vi "Handle URL.vi"(8 "error in (no error)":errorcluster, 10 "URL":string, 11 "FTP in":refnum<class "FTP.lvclass">) -> (0 "error out":errorcluster, 1 "directory":string, 2 "address":string, 3 "FTP out":refnum<class "FTP.lvclass">)   [LabVIEW 2017, in "FTP.lvlib" / "FTP.lvclass"]
uses:
  FTP.lvclass
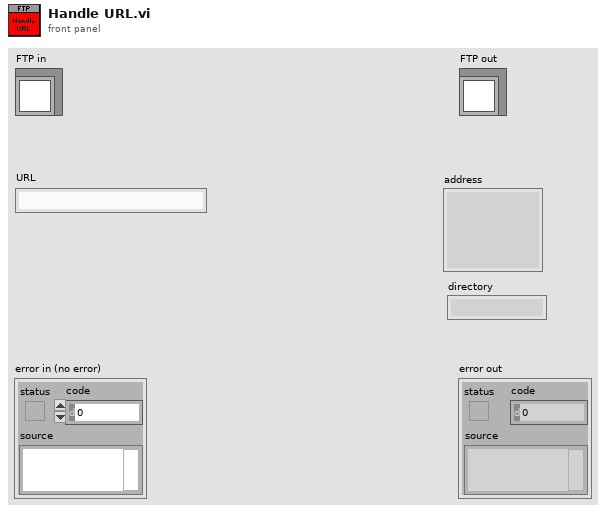
[diagram p1: front panel]
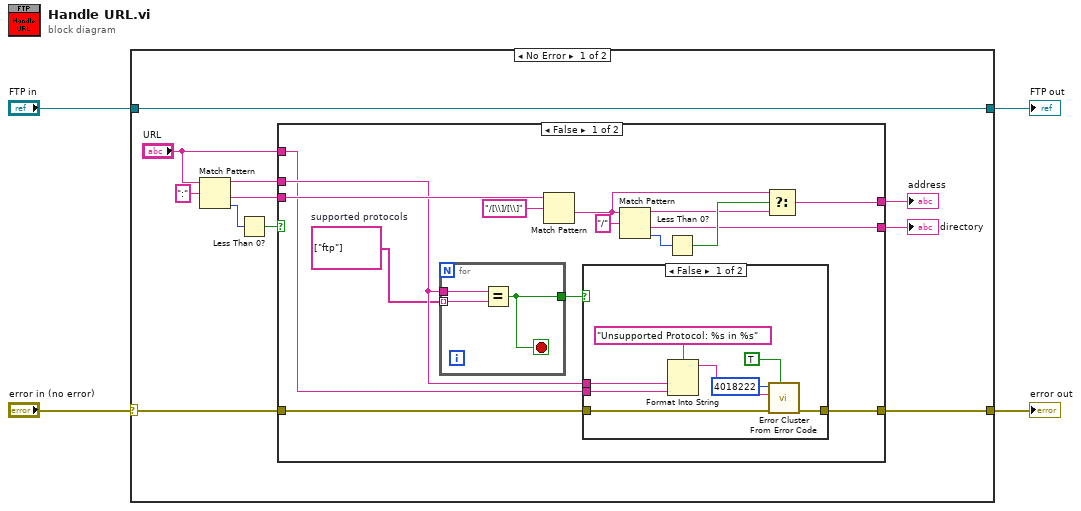
[diagram p0: block diagram]
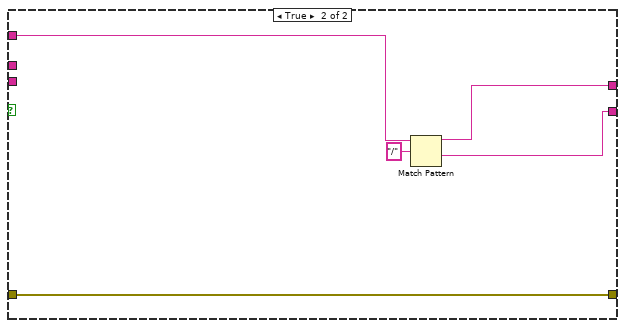
[diagram p3: hidden frame]
diagram:
  n1 = case shown="No Error" "error in (no error)" {
    selector: "error in (no error)" -> [w7 w49]
    tunnel: [w6 w49] -> w3
    tunnel: [w15 w48] -> w1
    tunnel: "FTP in" -> [w15 w48]
    frame No Error {
      n2 = Match Pattern(string="URL", regular expression=":") -> (before substring=w8:string, after substring=w12:string, offset past match=w13:i32)  [unwired: 1 in, 1 out]
      n3 = Less Than 0?(x=w13) -> (x < 0?=w10:bool)
      n4 = case shown="False" w10 {
        tunnel: w12 -> [w30 _]
        tunnel: [w18 w43] -> w11
        tunnel: "URL" -> [w25 w45]
        tunnel: w8 -> [w26 _]
        tunnel: w7 -> [w28 w47]
        tunnel: [w27 w47] -> w6
        tunnel: [w16 w44] -> w5
        frame False {
          w24 = string[] ["ftp"]  # supported protocols
          n5 = for {
            tunnel: w26 -> [w33]
            tunnel: w24 -> [w32] mode=indexing
            tunnel: [w31] -> w23
            stop <- w31 stop-if-true
            n6 = Equal?(x=w33, y=w32) -> (x = y?=w31:bool)
          }
          n7 = Match Pattern(string=w30, regular expression="/[\\]/[\\]") -> (after substring=w20:string)  [unwired: 1 in, 3 out]
          n8 = case shown="False" w23 {
            tunnel: w28 -> [w41 w42]
            tunnel: [w40 w42] -> w27
            tunnel: w26 -> [w38 _]
            tunnel: w25 -> [w35 _]
            frame False {
              n9 = Format Into String(format string="Unsupported Protocol: %s in %s", w38, w35) -> (resulting string=w36:string)  [unwired: 2 in, 1 out]
              n10 = call <vilib>:"Error Cluster From Error Code.vi"("show call chain? (False)"=TRUE, "error in (no error)"=w41, "error message (\"\")"=w36, "error code (0)"=4018222) -> ("error out"=w40:errorcluster)  [unwired: 5 in]
            }
            frame True {
            }
          }
          n11 = Match Pattern(string=w20, regular expression="/") -> (before substring=w17:string, after substring=w16:string, offset past match=w21:i32)  [unwired: 1 in, 1 out]
          n12 = Less Than 0?(x=w21) -> (x < 0?=w19:bool)
          n13 = Select(t=w20, s=w19, f=w17) -> (s? t:f=w18:string)
        }
        frame True {
          n14 = Match Pattern(string=w45, regular expression="/") -> (before substring=w43:string, after substring=w44:string)  [unwired: 1 in, 2 out]
        }
      }
      "address" <- w11
      "directory" <- w5
    }
    frame Error {
    }
  }
  "error out" <- w3
  "FTP out" <- w1
